vi "AverageAngleA.vi"(1 "Input":dbl) -> ()   [LabVIEW 2016]
uses:
  Robot Global Data.vi
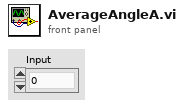
[diagram p1: front panel]
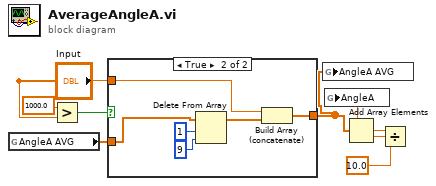
[diagram p0: block diagram]
diagram:
  n1 = global read "Robot Global Data.vi" "AngleA AVG"() -> (w5:dbl[])
  n2 = Greater?(x=1000.0, y="Input") -> (0:w6:bool)
  n3 = case shown="True" w6 {
    tunnel: w5 -> [w9 w13]
    tunnel: [w9 w11] -> w1
    tunnel: "Input" -> [_ w10]
    frame False {
    }
    frame True {
      n4 = Delete From Array(array=w13, length=1, index=9) -> (array with subset deleted=w12:dbl[])  [unwired: 1 out]
      n5 = Build Array (concatenate)(w10, w12) -> (w11:dbl[])
    }
  }
  n6 = global write "Robot Global Data.vi" "AngleA AVG"(w1) -> ()
  n7 = Add Array Elements(numeric array=w1) -> (sum=w8:dbl)
  n8 = Divide(x=w8, y=10.0) -> (x/y=w3:dbl)
  n9 = global write "Robot Global Data.vi" "AngleA"(w3) -> ()
